vi "662xA Set Mask Register.vi"(0 "VISA resource name":refnum<visa-resource-name>, 1 "unregulated mode (F:off)":bool, 2 "overtemperature (F:off)":bool, 3 "overvoltage (F:off)":bool, 5 "channel (1)":u8=1 min=1 max=4 step=1, 7 "coupled parameter (F:off)":bool, 9 "overcurrent (F:off)":bool, 11 "error in (no error)":errorcluster, 12 "-cc mode (F:off)":bool, 13 "+cc mode (F:off)":bool, 14 "cv mode (F:off)":bool) -> (4 "VISA resource name out":refnum<visa-resource-name>, 15 "error out":errorcluster)   [LabVIEW 2020, in "Agilent 6XXX Series.lvlib"]
doc: "This function sets the mask register which specifies which bits in the status register are enabled to set bits in the fault register. Basically, this function allows the operator to define which conditions are fault conditions."
uses:
  <instrlib>/Agilent 6XXX Series/Agilent 6XXX Series.lvlib
panel:
  # "HP662XA series only"
  # "Set Mask for.."
  # "on\noff"
  # "on\noff"
  # "on\noff"
  # "on\noff"
  # "on\noff"
  # "on\noff"
  # "on\noff"
  # "on\noff"
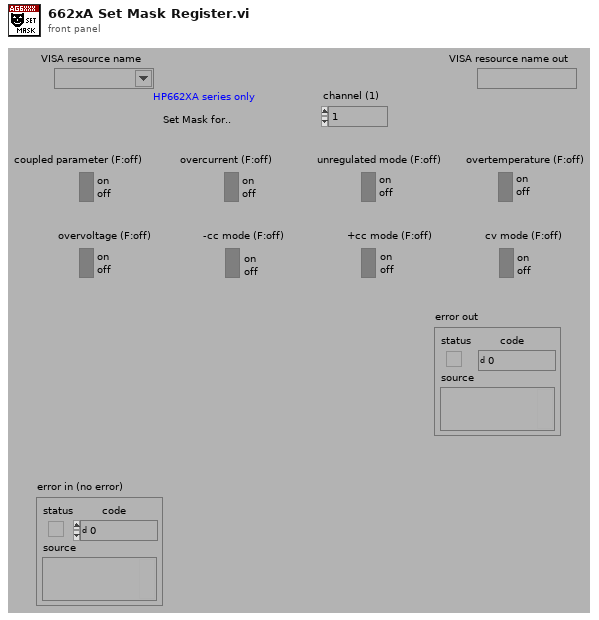
[diagram p1: front panel]
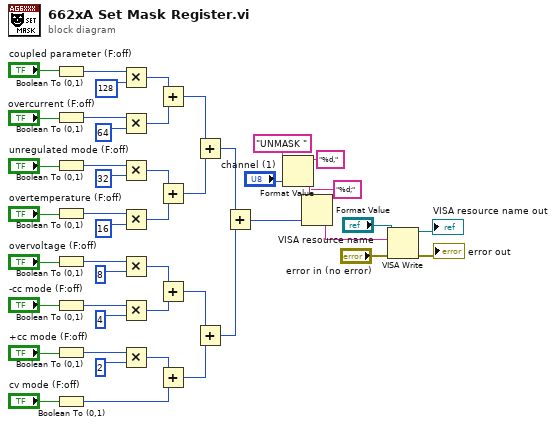
[diagram p0: block diagram]
diagram:
  n1 = Boolean To (0,1)(Boolean="coupled parameter (F:off)") -> (0, 1=w39:i16)
  n2 = Boolean To (0,1)(Boolean="overcurrent (F:off)") -> (0, 1=w38:i16)
  n3 = Boolean To (0,1)(Boolean="unregulated mode (F:off)") -> (0, 1=w37:i16)
  n4 = Boolean To (0,1)(Boolean="overtemperature (F:off)") -> (0, 1=w36:i16)
  n5 = Boolean To (0,1)(Boolean="overvoltage (F:off)") -> (0, 1=w35:i16)
  n6 = Boolean To (0,1)(Boolean="-cc mode (F:off)") -> (0, 1=w34:i16)
  n7 = Boolean To (0,1)(Boolean="+cc mode (F:off)") -> (0, 1=w33:i16)
  n8 = Boolean To (0,1)(Boolean="cv mode (F:off)") -> (0, 1=w19:i16)
  n9 = Multiply(x=w39, y=i16 128) -> (x*y=w12:i16)
  n10 = Multiply(x=w38, y=i16 64) -> (x*y=w13:i16)
  n11 = Multiply(x=w37, y=i16 32) -> (x*y=w14:i16)
  n12 = Multiply(x=w36, y=i16 16) -> (x*y=w15:i16)
  n13 = Multiply(x=w35, y=i16 8) -> (x*y=w16:i16)
  n14 = Multiply(x=w34, y=i16 4) -> (x*y=w17:i16)
  n15 = Multiply(x=w33, y=i16 2) -> (x*y=w18:i16)
  n16 = Add(x=w12, y=w13) -> (x+y=w11:i16)
  n17 = Add(x=w14, y=w15) -> (x+y=w10:i16)
  n18 = Add(x=w16, y=w17) -> (x+y=w8:i16)
  n19 = Add(x=w18, y=w19) -> (x+y=w9:i16)
  n20 = Add(x=w11, y=w10) -> (x+y=w25:i16)
  n21 = Add(x=w8, y=w9) -> (x+y=w7:i16)
  n22 = Add(x=w25, y=w7) -> (x+y=w2:i16)
  n23 = Format Value(string ("")="UNMASK ", format string="%d,", value (0)="channel (1)") -> (output string=w6:string)
  n24 = Format Value(string ("")=w6, format string="%d;", value (0)=w2) -> (output string=w1:string)
  n25 = VISA Write(VISA resource name="VISA resource name", write buffer=w1, error in (no error)="error in (no error)") -> (VISA resource name out=→"VISA resource name out":refnum<visa-resource-name>, error out=→"error out":errorcluster)  [unwired: 1 out]
